vi "OpenLatestFileAndReadLines.vi"(2 "No. of lines to read":i32, 3 "pattern":string, 4 "path":path) -> (1 "Lines":string[](array[string]))   [LabVIEW 2015]
panel:
  out "filenames 2":string[](array[string])
  out "Latest file: 2":path
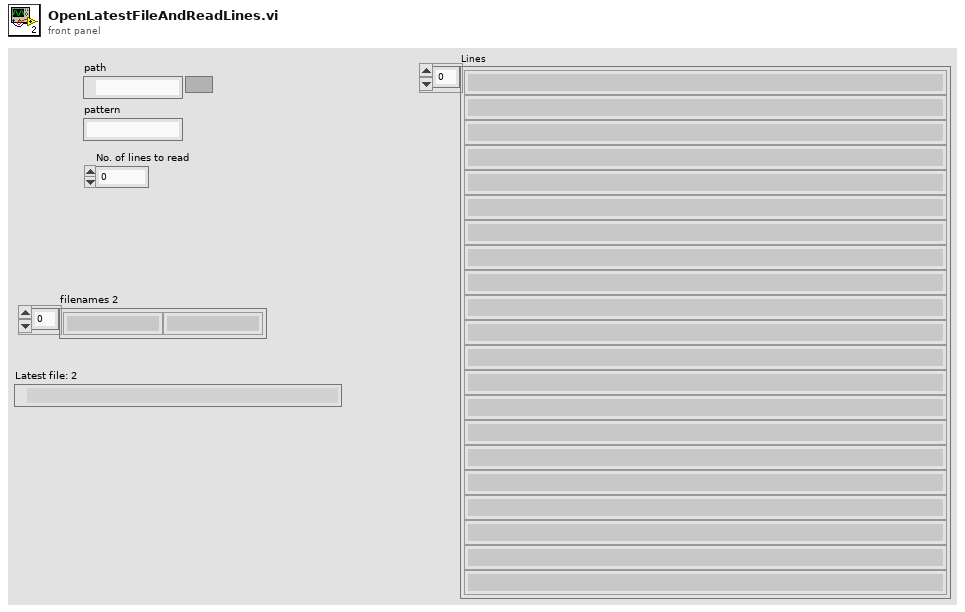
[diagram p1: front panel]
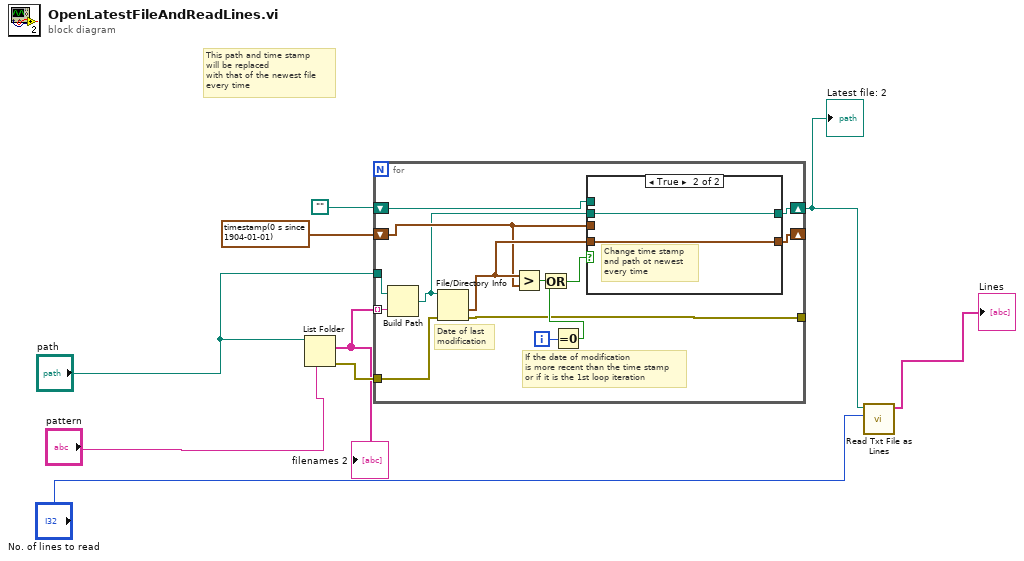
[diagram p0: block diagram]
diagram:
  # "This path and time stamp\nwill be replaced\nwith that of the newest file \nevery time"
  n1 = List Folder(path="path", pattern="pattern") -> (filenames=w4:string[], error out=w6:errorcluster)  [unwired: 2 in, 2 out]
  "filenames 2" <- w4
  n2 = for {
    tunnel: w4 -> [w13] mode=indexing
    tunnel: "path" -> [w23]
    shift-right: [w18] -> _
    shift-left: timestamp(0 s since 1904-01-01) ("last mod 2") -> [w16]
    shift-right: [w17] -> w7
    shift-left: path "" -> [w14]
    tunnel: w6 -> [w11]
    tunnel: [w10] -> _
    i -> [w21]
    # "If the date of modification\nis more recent than the time stamp\nor if it is the 1st loop iteration"
    # "Date of last\nmodification"
    n3 = Build Path(base path=w23, name or relative path=w13) -> (appended path=w12:path)
    n4 = File/Directory Info(path=w12, error in=w11) -> (last mod=w19:timestamp, error out=w10:errorcluster)  [unwired: 5 out]
    n5 = Greater?(x=w19, y=w16) -> (0:w22:bool)
    n6 = Equal To 0?(x=w21) -> (x = 0?=w20:bool)
    n7 = Or(x=w22, y=w20) -> (x .or. y?=w15:bool)
    n8 = case shown="True" w15 {
      tunnel: w16 -> [w25 _]
      tunnel: w19 -> [_ w27]
      tunnel: w12 -> [_ w26]
      tunnel: [w24 w26] -> w17
      tunnel: w14 -> [w24 _]
      tunnel: [w25 w27] -> w18
      frame False {
        # "save the same time stamp \nand path as before"
      }
      frame True {
        # "Change time stamp\nand path ot newest \nevery time"
      }
    }
  }
  "Latest file: 2" <- w7
  n9 = call "Read Txt File as Lines.vi"("Lines to Read"="No. of lines to read", "file path (use dialog)"=w7) -> ("Lines"=→"Lines":string[])  [unwired: 8 in, 1 out]
